vi "Pick Up and Rotate.vi"(0 "Degrees":dbl=90.0 format="%#_13g", 1 "Distance (ft)":dbl=7.0 format="%#_13g", 2 "Clockwise?":bool) -> ()   [LabVIEW 2014]
panel:
  in  "Divisor":dbl=50.0 format="%#_13g"
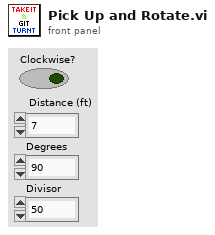
[diagram p1: front panel]
types:
  T1 = enum16{"Move Forward", "Move Backward", "Strafe Right", "Strafe Left"}
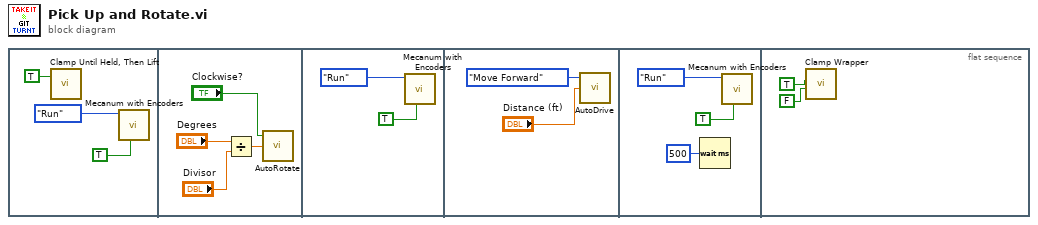
[diagram p0: block diagram]
diagram:
  n1 = flat-sequence {
    frame #0 {
      n2 = call "Clamp Until Held, Then Lift.vi"("Clamp + Lift"=TRUE) -> ()  [unwired: 2 in]
      n3 = call "Mecanum with Encoders.vi"("Reset"=TRUE, "Mode"=enum8{"Start", "Run", "Finish"}."Run") -> ()  [unwired: 8 in, 1 out]
    }
    frame #1 {
      n4 = Divide(x="Degrees", y="Divisor") -> (x/y=w4:dbl)
      n5 = call "AutoRotate.vi"("Degrees"=w4, "Clockwise?"="Clockwise?") -> ()  [unwired: 1 in, 1 out]
    }
    frame #2 {
      n6 = call "Mecanum with Encoders.vi"("Reset"=TRUE, "Mode"=enum8{"Start", "Run", "Finish"}."Run") -> ()  [unwired: 8 in, 1 out]
    }
    frame #3 {
      n7 = call "AutoDrive.vi"("Distance (ft)"="Distance (ft)", "Direction"=T1."Move Forward") -> ()  [unwired: 1 in, 1 out]
    }
    frame #4 {
      n8 = Wait (ms)(milliseconds to wait=u32 500) -> ()  [unwired: 1 out]
      n9 = call "Mecanum with Encoders.vi"("Reset"=TRUE, "Mode"=enum8{"Start", "Run", "Finish"}."Run") -> ()  [unwired: 8 in, 1 out]
    }
    frame #5 {
      n10 = call "Clamp Wrapper.vi"("In"=FALSE, "Out"=TRUE) -> ()  [unwired: 2 in]
    }
  }
